vi "Update State Data.vi"(8 "error in (no error)":errorcluster, 9 "Data":variant, 10 "Argument":string, 11 "State Data":T1={"Core"={"Current VI Reference"=refnum, "Close Panel on Exit?"=FALSE}, "FP Refs"={"VI Tree"=refnum, "Window Title"=refnum, "Same as VI?"=refnum, "VI Desc"=refnum, "Help Path"=refnum, "Help Tag"=refnum, "Controls"=refnum}, "New VI Data"=[], "Saved VI Data"=[], "Current Path"=path "", "FP"={"Selected VI Data"=0, "Help Path"="", "Help Tag"="", "Help URL"="", "Help Type"=enum."Local Help File", "VI Desc"="", "Controls"=[], "Window Title"="", "Same Title?"=FALSE, "VI Tree Value"=""}, "Config Path"=path "", "Config"={"Copyright Path"=path "", "Recent Folders"=[], "Recent Files"=[], "Recent Filters"=[], "Abbreviate Names?"=FALSE, "Format Bold Tags?"=FALSE, "Show ConPane Only?"=FALSE, "Confirm Save?"=FALSE, "Confirm Revert?"=FALSE, "Confirm Save All?"=FALSE, "Confirm Revert All?"=FALSE, "Confirm Exit?"=FALSE, "Flat View?"=FALSE}, "Desc Selection"={"Selection Start"=0, "Selection End"=0}, "Displayed Indices"=[], "Filter"={"Filter Column"=enum."Description", "Filter Type"=enum."Contains", "Filter Value"="", "New Data?"=FALSE, "Enabled?"=FALSE}, "Sort"={"Sort Column"=enum."Description", "Ascending?"=FALSE, "Enabled?"=FALSE}, "Tree Map"=refnum, "VI Blacklist"={}}) -> (0 "error out":errorcluster, 3 "State Data out":T1={"Core"={"Current VI Reference"=refnum, "Close Panel on Exit?"=FALSE}, "FP Refs"={"VI Tree"=refnum, "Window Title"=refnum, "Same as VI?"=refnum, "VI Desc"=refnum, "Help Path"=refnum, "Help Tag"=refnum, "Controls"=refnum}, "New VI Data"=[], "Saved VI Data"=[], "Current Path"=path "", "FP"={"Selected VI Data"=0, "Help Path"="", "Help Tag"="", "Help URL"="", "Help Type"=enum."Local Help File", "VI Desc"="", "Controls"=[], "Window Title"="", "Same Title?"=FALSE, "VI Tree Value"=""}, "Config Path"=path "", "Config"={"Copyright Path"=path "", "Recent Folders"=[], "Recent Files"=[], "Recent Filters"=[], "Abbreviate Names?"=FALSE, "Format Bold Tags?"=FALSE, "Show ConPane Only?"=FALSE, "Confirm Save?"=FALSE, "Confirm Revert?"=FALSE, "Confirm Save All?"=FALSE, "Confirm Revert All?"=FALSE, "Confirm Exit?"=FALSE, "Flat View?"=FALSE}, "Desc Selection"={"Selection Start"=0, "Selection End"=0}, "Displayed Indices"=[], "Filter"={"Filter Column"=enum."Description", "Filter Type"=enum."Contains", "Filter Value"="", "New Data?"=FALSE, "Enabled?"=FALSE}, "Sort"={"Sort Column"=enum."Description", "Ascending?"=FALSE, "Enabled?"=FALSE}, "Tree Map"=refnum, "VI Blacklist"={}})   [LabVIEW 2020, in "VI Properties Editor.lvlib"]
doc: "Updates one or more elements of <B>State Data</B> based on <B>Argument</B> and <B>Data</B>."
uses:
  VI Properties Editor.lvlib
  Tree Map/Tree Map/Tree Map.lvclass
  <vilib>/ErrorRing/Error Ring.xnode
  3573416a-ab14-40fa-8eb1-e5c23e8662a1.vi
  6c3ab29c-e086-46da-822f-1f7a3bdde8cc.vi
  CTLs/Column Name.ctl
  CTLs/Filter Type.ctl
  c05ae38d-f8ec-456d-8819-95a6d1f6576e.vi
  <vilib>/Utility/error.llb/Error Cluster From Error Code.vi
  <vilib>/picture/picture.llb/imagedata.ctl
  CTLs/VI Properties.ctl
  CTLs/Control Properties.ctl
  CTLs/VI Data.ctl
  CTLs/Main Front Panel Controls.ctl
  CTLs/Config.ctl
  <vilib>/Utility/miscctls.llb/LVSelectionTypeDef.ctl
  CTLs/Filter Info.ctl
  CTLs/Main References.ctl
  CTLs/Main State Data.ctl
  CTLs/Sort Info.ctl
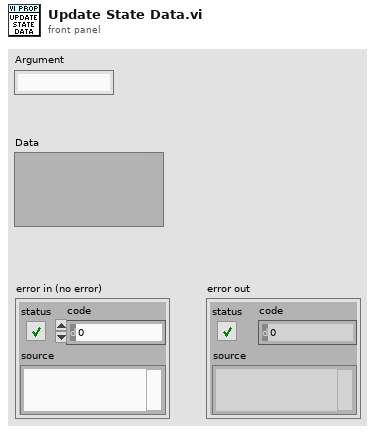
[diagram p1: front panel]
types:
  T1 = typedef "VI Properties Editor.lvlib/Main State Data.ctl" = cluster{"Core":cluster{"Current VI Reference":refnum<vi>, "Close Panel on Exit?":bool}, "FP Refs":T2, "New VI Data":T3[], "Saved VI Data":T3[], "Current Path":path, "FP":T7, "Config Path":path, "Config":T8, "Desc Selection":T12, "Displayed Indices":i32[], "Filter":T9, "Sort":T13, "Tree Map":refnum<class "Tree Map.lvclass">, "VI Blacklist":set{string}}
  T2 = typedef "VI Properties Editor.lvlib/Main References.ctl" = cluster{"VI Tree":refnum<vi>, "Window Title":refnum<vi>, "Same as VI?":refnum<vi>, "VI Desc":refnum<vi>, "Help Path":refnum<vi>, "Help Tag":refnum<vi>, "Controls":refnum<vi>}
  T3 = typedef "VI Properties Editor.lvlib/VI Data.ctl" = cluster{"VI":T4, "Ctl Properties":T6[], "Hierarchy":string}
  T4 = typedef "VI Properties Editor.lvlib/VI Properties.ctl" = cluster{"Name":string, "Path":path, "Type":enum32{"invalid VI type", "Standard VI", "Control VI", "Global VI", "Polymorphic VI", "Configuration VI", "SubSystem", "Facade VI", "Method VI", "Statechart Diagram VI"}, "Window Title":string, "Description":string, "Help Path":path, "Help Tag":string, "Help Web URL":string, "Use Web URL?":bool, "Custom Title?":bool, "Allow Debugging?":bool, "Reentrant?":bool, "Inlined?":bool, "Reentrancy Type":enum16{"Share clones between instances", "Preallocate clone for each instance"}, "Priority":enum32{"invalid priority", "background priority", "normal priority", "above normal priority", "high priority", "time critical priority", "subroutine"}, "Preferred Exec System":enum32{"invalid execution system", "user interface", "standard", "instrument i/o", "data acquisition", "other 1", "other 2", "same as caller"}, "Auto Error Handling?":bool, "Run When Opened?":bool, "Suspend When Called?":bool, "Conpane Img":T5}
  T5 = typedef "imagedata.ctl" = cluster{"image type":i32, "image depth":i32, "image":u8[], "mask":u8[], "colors":u32[], "Rectangle":cluster{"left":i16, "top":i16, "right":i16, "bottom":i16}}
  T6 = typedef "VI Properties Editor.lvlib/Control Properties.ctl" = cluster{"UID":i32, "Name":string, "Caption":string, "Description":string, "Tip Strip":string, "Is Indicator?":bool, "Is on ConPane?":bool}
  T7 = typedef "VI Properties Editor.lvlib/Main Front Panel Controls.ctl" = cluster{"Selected VI Data":i32, "Help Path":string, "Help Tag":string, "Help URL":string, "Help Type":enum16{"Local Help File", "Web-based Help"}, "VI Desc":string, "Controls":string[][], "Window Title":string, "Same Title?":bool, "VI Tree Value":string}
  T8 = typedef "VI Properties Editor.lvlib/Config.ctl" = cluster{"Copyright Path":path, "Recent Folders":path[], "Recent Files":path[], "Recent Filters":T9[], "Abbreviate Names?":bool, "Format Bold Tags?":bool, "Show ConPane Only?":bool, "Confirm Save?":bool, "Confirm Revert?":bool, "Confirm Save All?":bool, "Confirm Revert All?":bool, "Confirm Exit?":bool, "Flat View?":bool}
  T9 = typedef "VI Properties Editor.lvlib/Filter Info.ctl" = cluster{"Filter Column":T10, "Filter Type":T11, "Filter Value":string, "New Data?":bool, "Enabled?":bool}
  T10 = typedef "VI Properties Editor.lvlib/Column Name.ctl" = enum16{"Name", "Path", "Type", "Window Title", "Description", "Help Path", "Help Tag", "Custom Title?", "Reentrancy", "Inlined?", "Help URL", "Help Type", "Allow Debugging?", "Auto Error Handling?", "Run When Opened?", "Suspend When Called?", "Priority", "Preferred Exec Sytem"}
  T11 = typedef "VI Properties Editor.lvlib/Filter Type.ctl" = enum16{"Contains", "Equals", "Starts with", "Ends with", "Does not contain", "Does not equal", "Is empty", "Is not empty"}
  T12 = typedef "LVSelectionTypeDef.ctl" = cluster{"Selection Start":u32, "Selection End":u32}
  T13 = typedef "VI Properties Editor.lvlib/Sort Info.ctl" = cluster{"Sort Column":T10, "Ascending?":bool, "Enabled?":bool}
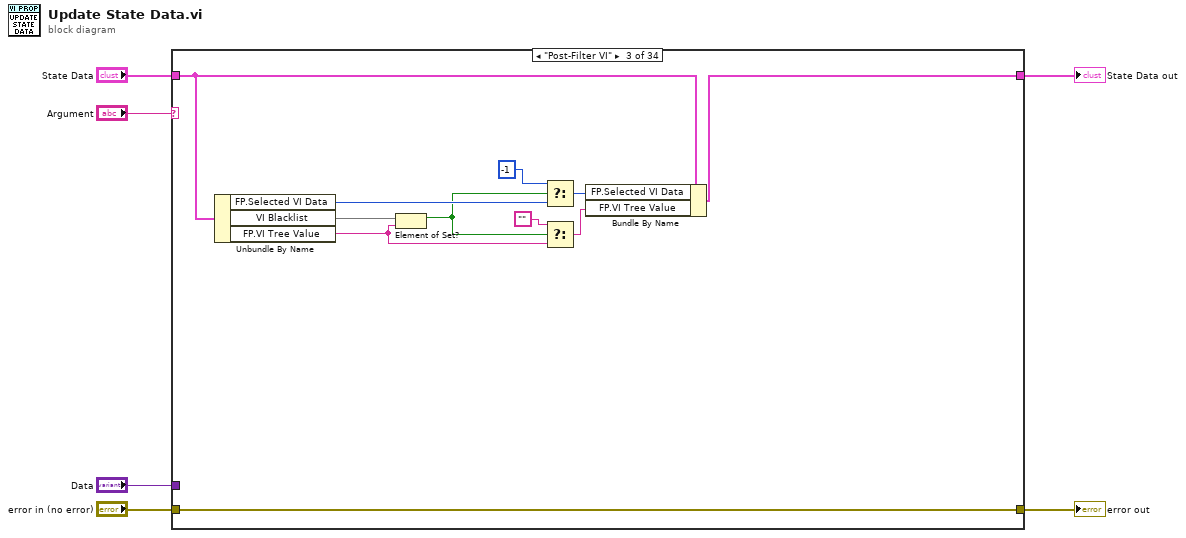
[diagram p0: block diagram]
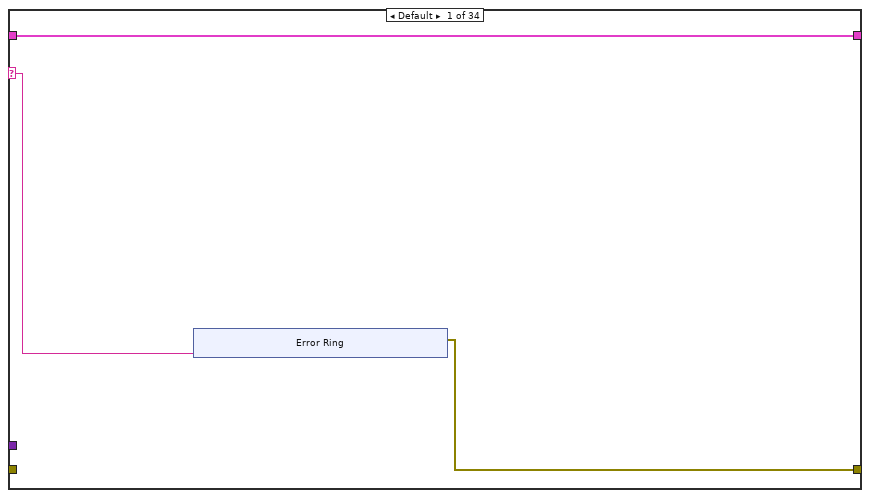
[diagram p2: hidden frame]
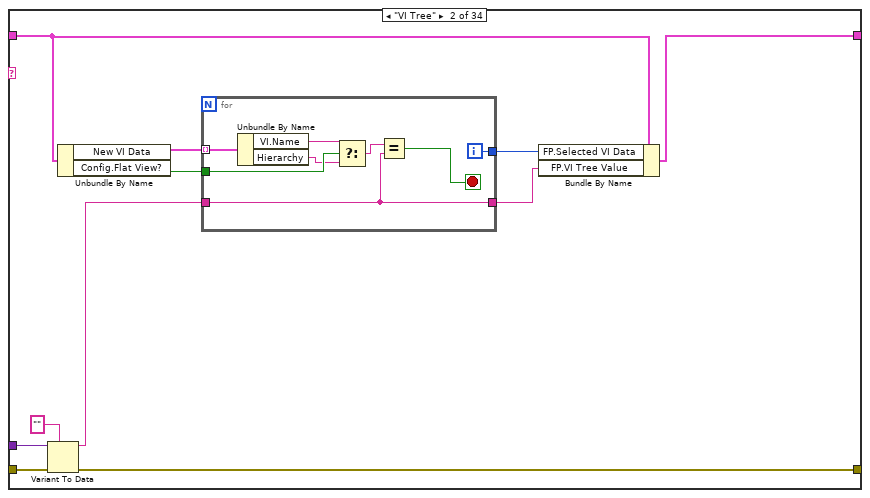
[diagram p3: hidden frame]
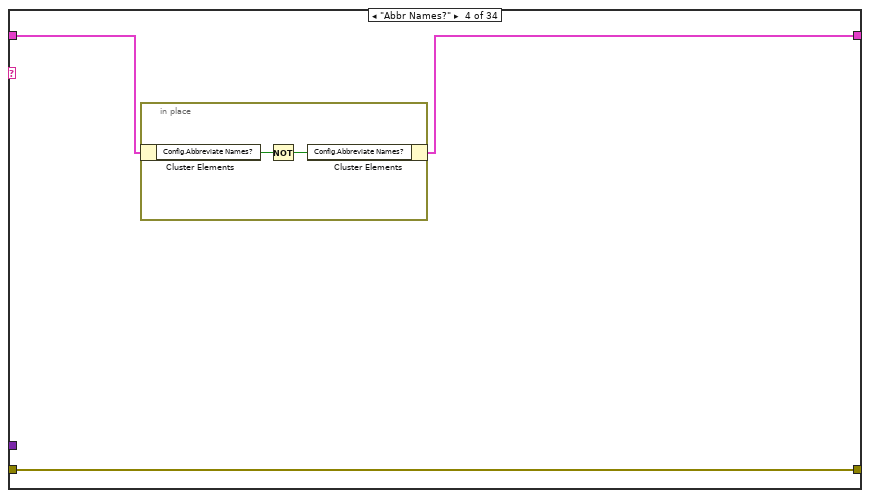
[diagram p4: hidden frame]
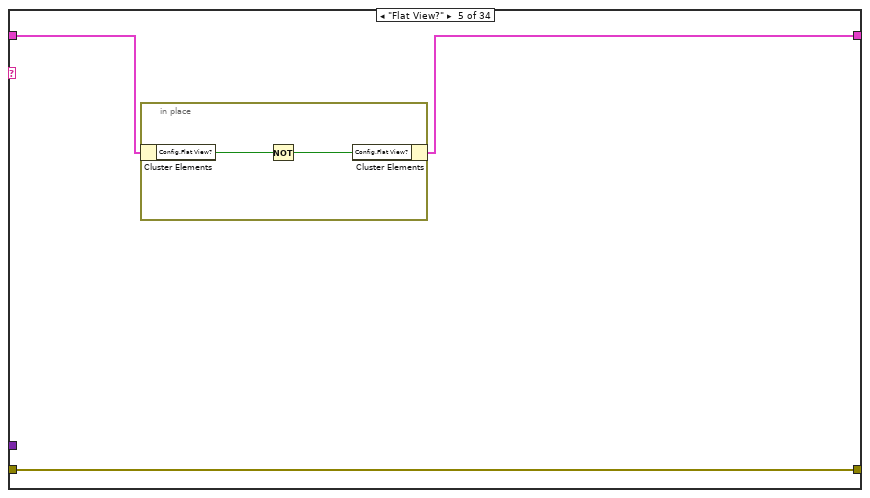
[diagram p5: hidden frame]
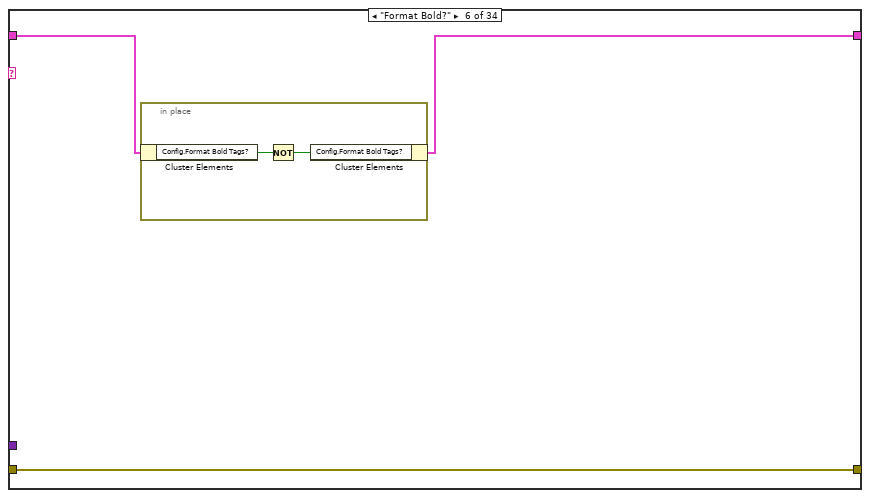
[diagram p6: hidden frame]
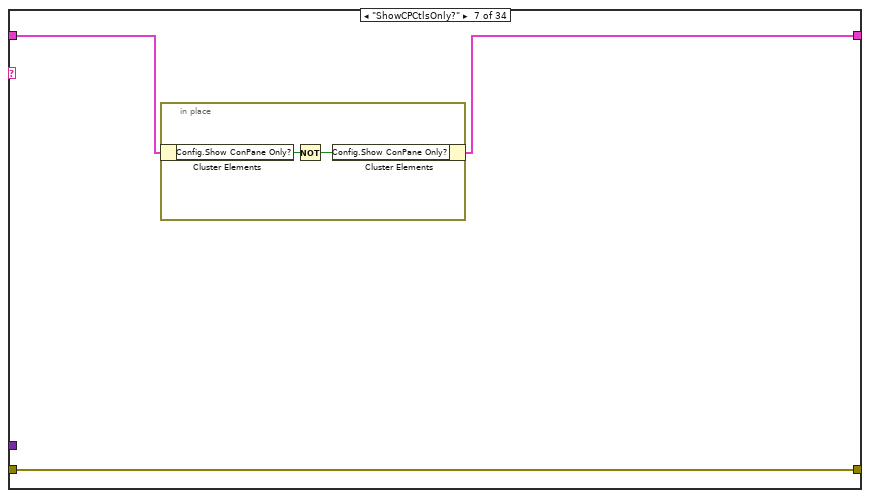
[diagram p7: hidden frame]
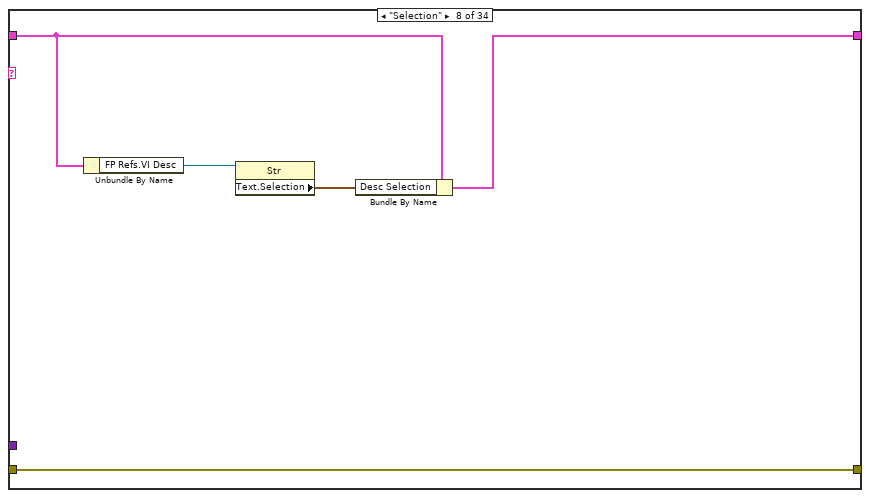
[diagram p8: hidden frame]
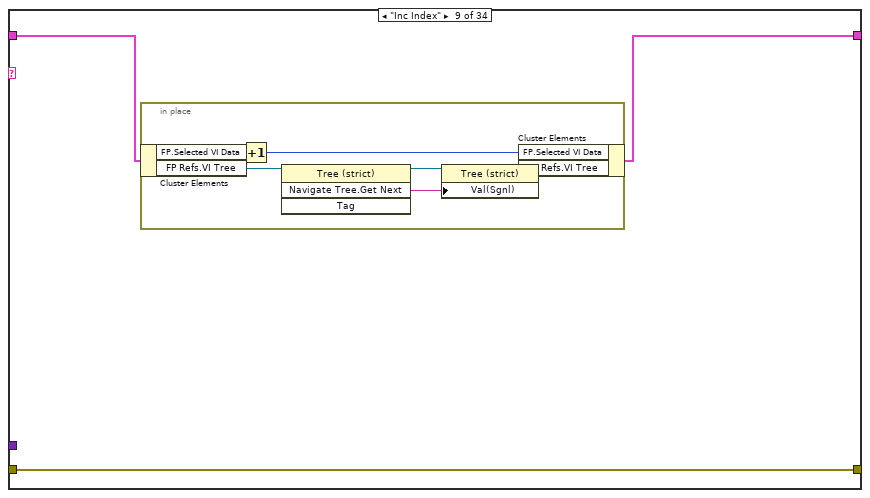
[diagram p9: hidden frame]
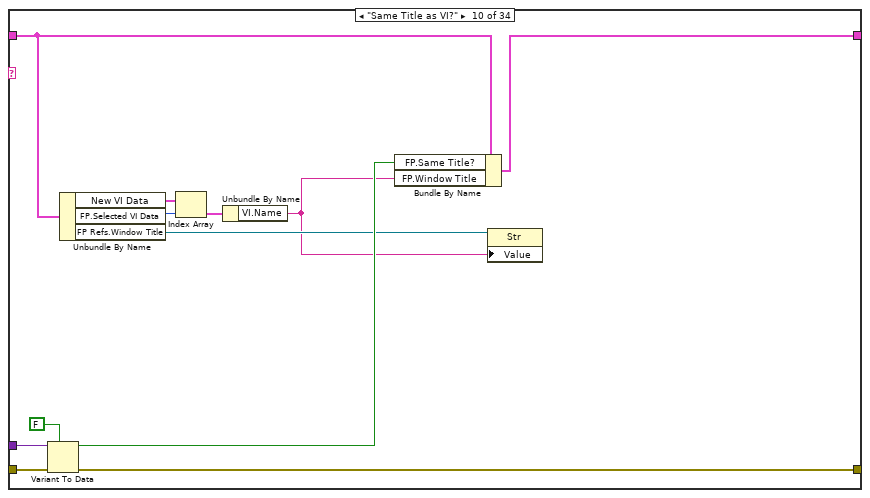
[diagram p10: hidden frame]
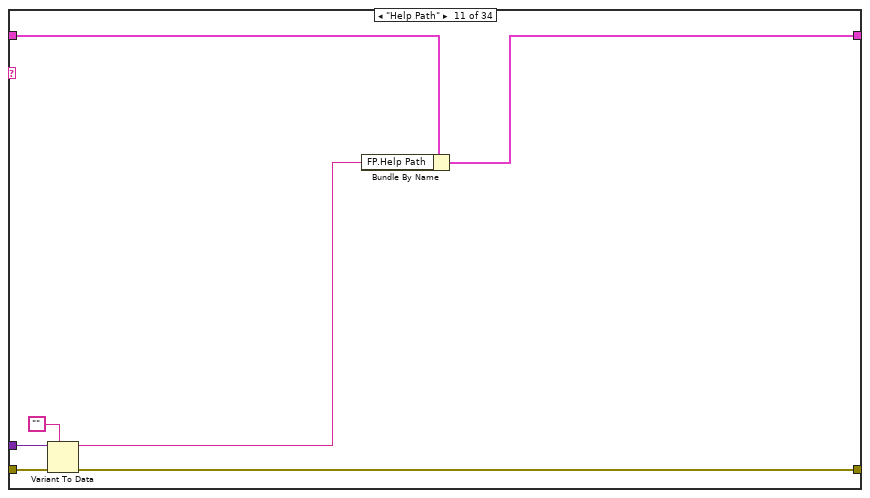
[diagram p11: hidden frame]
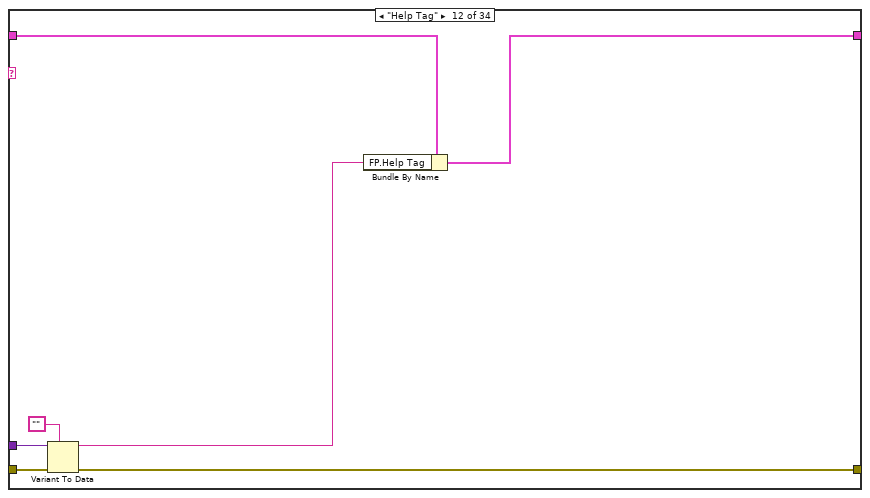
[diagram p12: hidden frame]
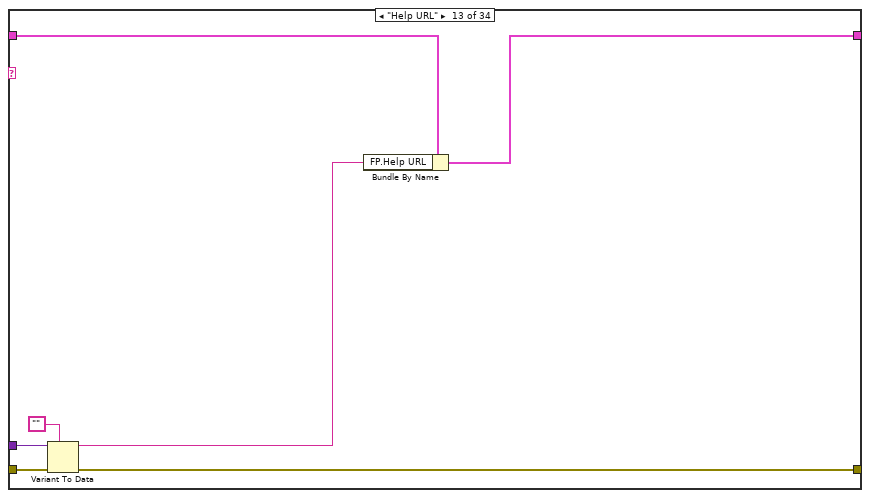
[diagram p13: hidden frame]
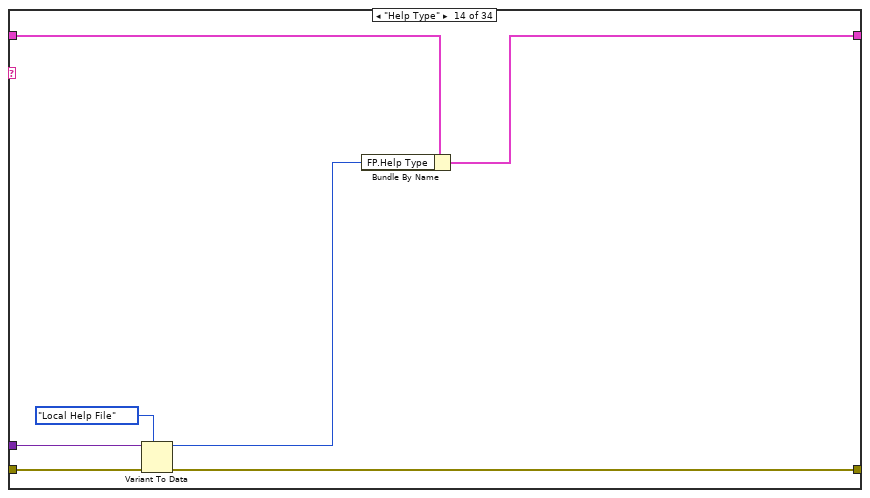
[diagram p14: hidden frame]
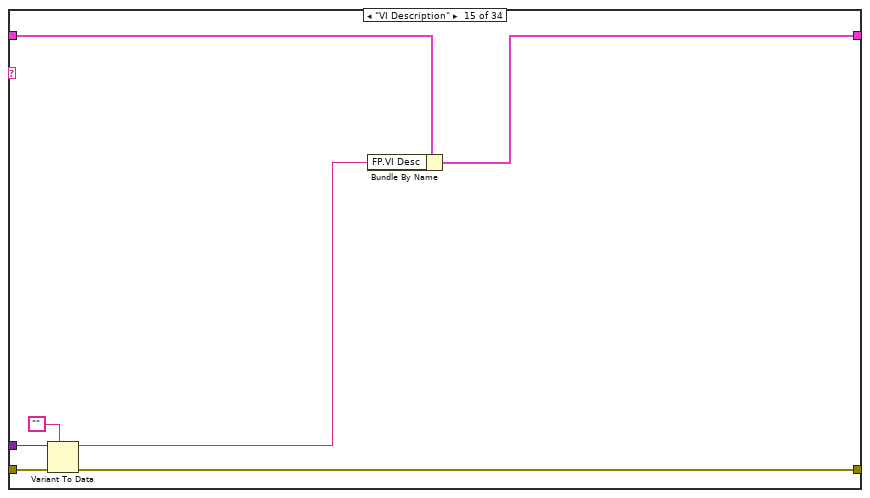
[diagram p15: hidden frame]
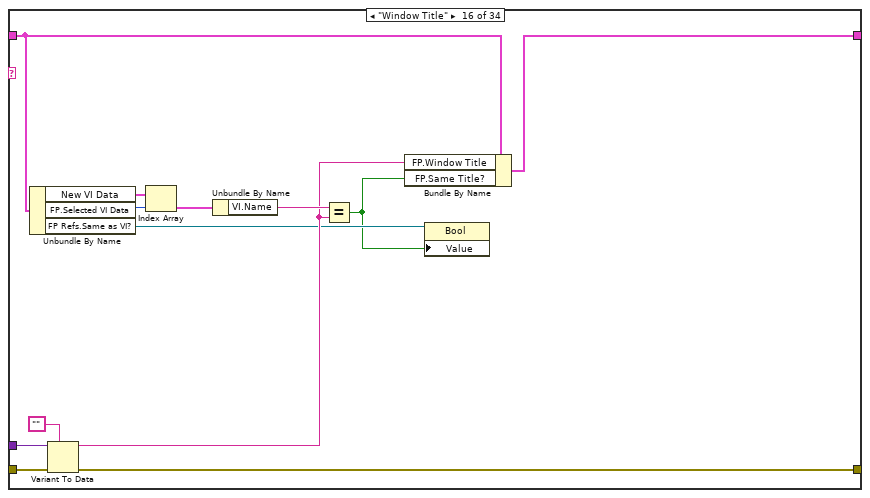
[diagram p16: hidden frame]
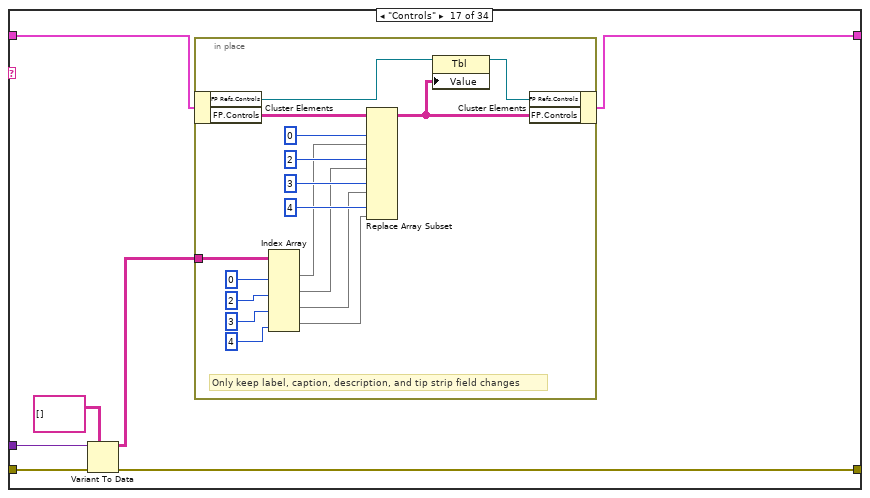
[diagram p17: hidden frame]
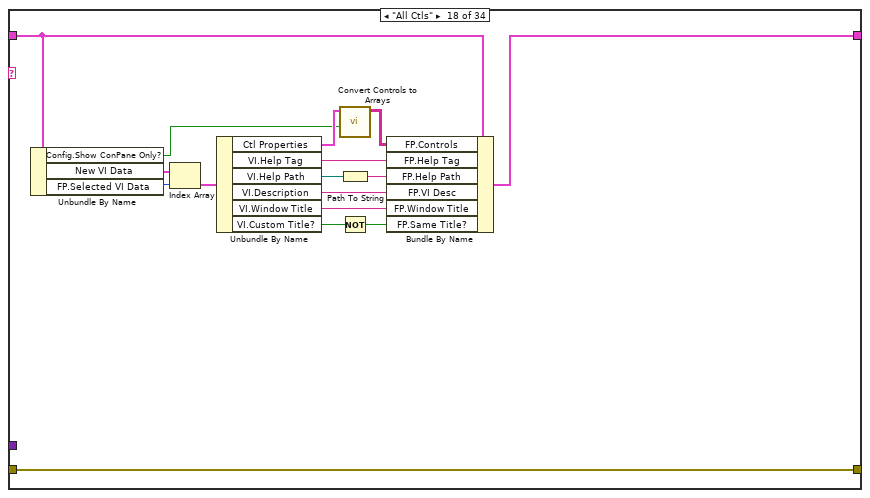
[diagram p18: hidden frame]
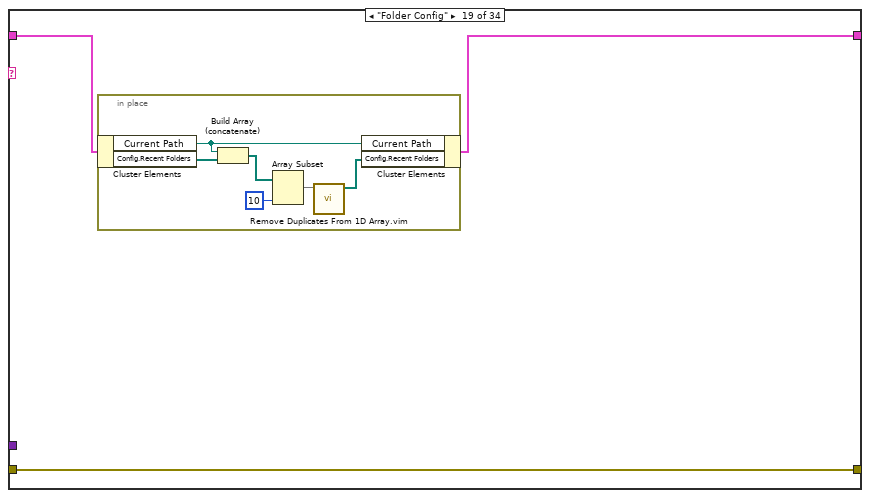
[diagram p19: hidden frame]
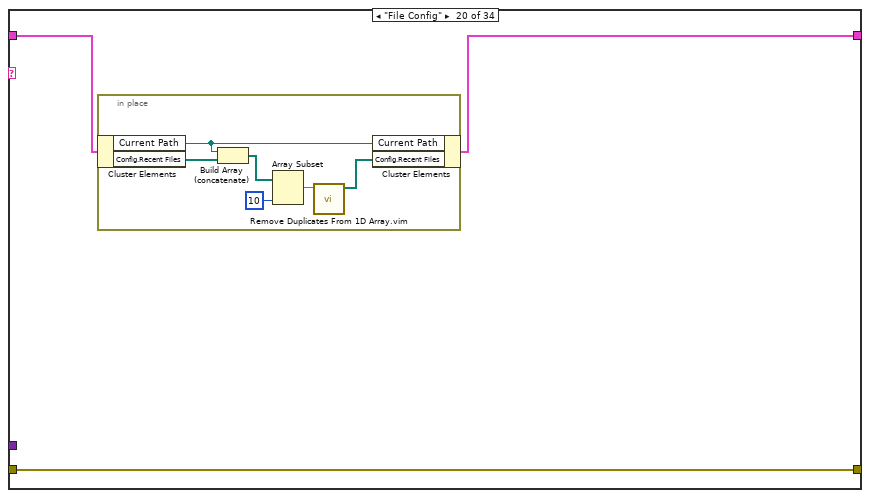
[diagram p20: hidden frame]
diagram:
  n1 = case shown="\"Post-Filter VI\"" "Argument" {
    selector: "Argument" -> [w8 _ _ _ _ _ _ _ _ _ _ _ _ _ _ _ _ _ _ _ _ w214 w224 w234 w248 w258 _ _ _ _ w293 _ _ _]
    tunnel: "error in (no error)" -> [_ w27 w44 w49 w54 w59 w64 w71 w74 w92 w99 w106 w113 w120 w127 w140 w147 w178 w183 w192 w201 w216 w226 w236 w250 w260 w266 w272 w279 w284 w295 w300 w305 w310]
    tunnel: "State Data" -> [w9 w22 w45 w48 w53 w58 w63 w68 w73 w83 w96 w103 w110 w118 w124 w133 w143 w179 w181 w190 w199 w210 w220 w230 w244 w254 w264 w270 w277 w282 w290 w298 w303 w308]
    tunnel: "Data" -> [_ w26 _ _ _ _ _ _ _ w91 w98 w105 w112 w119 w126 w139 w146 _ _ _ _ _ _ _ _ _ _ _ _ _ _ _ _ _]
    tunnel: [w7 w24 w44 w49 w54 w59 w64 w71 w74 w88 w94 w101 w108 w117 w122 w137 w145 w178 w183 w192 w201 w216 w226 w236 w250 w260 w266 w272 w279 w284 w295 w300 w305 w310] -> w1
    tunnel: [w9 w23 w46 w47 w52 w57 w62 w69 w72 w87 w93 w100 w107 w116 w121 w136 w141 w180 w182 w191 w200 w215 w225 w235 w249 w259 w265 w271 w278 w283 w294 w299 w304 w309] -> w5
    frame Default {
      n2 = xnode "Error Ring"("parameter 0"=w8) -> ("error out"=w7:errorcluster)
    }
    frame "VI Tree" {
      n3 = Variant To Data(error in=w27, type="", Variant=w26) -> (data=w19:string, error out=w24:errorcluster)
      n4 = Unbundle By Name(w22) -> ("New VI Data"=w21:T3[], "Config.Flat View?"=w17:bool)
      n5 = for {
        tunnel: w21 -> [w35] mode=indexing
        tunnel: [w34] -> w20
        tunnel: w19 -> [w32]
        tunnel: [w32] -> w18
        tunnel: w17 -> [w30]
        i -> [w34]
        stop <- w33 stop-if-true
        n6 = Unbundle By Name(w35) -> ("VI.Name"=w29:string, "Hierarchy"=w28:string)
        n7 = Select(t=w29, s=w30, f=w28) -> (s? t:f=w31:string)
        n8 = Equal?(x=w31, y=w32) -> (x = y?=w33:bool)
      }
      n9 = Bundle By Name(cluster=w22, "FP.Selected VI Data"=w20, "FP.VI Tree Value"=w18) -> (w23:T1)
    }
    frame "Post-Filter VI" {
      n10 = Unbundle By Name(w45) -> ("FP.Selected VI Data"=w40:i32, "VI Blacklist"=w42:set{string}, "FP.VI Tree Value"=w36:string)
      n11 = Element of Set?(10:w36, 11:w42) -> (3:w39:bool)
      n12 = Select(t=-1, s=w39, f=w40) -> (s? t:f=w43:i32)
      n13 = Select(t="", s=w39, f=w36) -> (s? t:f=w38:string)
      n14 = Bundle By Name(cluster=w45, "FP.Selected VI Data"=w43, "FP.VI Tree Value"=w38) -> (w46:T1)
    }
    frame "Abbr Names?" {
      n15 = in-place {
        n16 = in-place-cluster #1(w48) -> ("Config.Abbreviate Names?"=w51:bool)
        n17 = Not(x=w51) -> (.not. x?=w50:bool)
        n18 = in-place-cluster #1("Config.Abbreviate Names?"=w50) -> (w47:T1)
      }
    }
    frame "Flat View?" {
      n19 = in-place {
        n20 = in-place-cluster #2(w53) -> ("Config.Flat View?"=w56:bool)
        n21 = Not(x=w56) -> (.not. x?=w55:bool)
        n22 = in-place-cluster #2("Config.Flat View?"=w55) -> (w52:T1)
      }
    }
    frame "Format Bold?" {
      n23 = in-place {
        n24 = in-place-cluster #3(w58) -> ("Config.Format Bold Tags?"=w61:bool)
        n25 = Not(x=w61) -> (.not. x?=w60:bool)
        n26 = in-place-cluster #3("Config.Format Bold Tags?"=w60) -> (w57:T1)
      }
    }
    frame "ShowCPCtlsOnly?" {
      n27 = in-place {
        n28 = in-place-cluster #4(w63) -> ("Config.Show ConPane Only?"=w66:bool)
        n29 = Not(x=w66) -> (.not. x?=w65:bool)
        n30 = in-place-cluster #4("Config.Show ConPane Only?"=w65) -> (w62:T1)
      }
    }
    frame "Selection" {
      n31 = Unbundle By Name(w68) -> ("FP Refs.VI Desc"=w67:refnum<vi>)
      n32 = property on="Property Node" class="Str"(reference=w67) -> ("Text.Selection"=w70:T12)  [unwired: 1 in, 2 out]
      n33 = Bundle By Name(cluster=w68, "Desc Selection"=w70) -> (w69:T1)
    }
    frame "Inc Index" {
      n34 = in-place {
        n35 = in-place-cluster #5(w73) -> ("FP.Selected VI Data"=w80:i32, "FP Refs.VI Tree"=w79:refnum<vi>)
        n36 = Increment(x=w80) -> (x+1=w77:i32)
        n37 = invoke class="Tree (strict)" method="Navigate Tree.Get Next"(reference=w79) -> (reference out=w78:refnum<vi>, "Navigate Tree:Get Next Item"=w75:string)  [unwired: 3 in, 2 out]
        n38 = property class="Tree (strict)"(reference=w78, "Val(Sgnl)"=w75) -> (reference out=w76:refnum<vi>)  [unwired: 1 in, 1 out]
        n39 = in-place-cluster #5("FP.Selected VI Data"=w77, "FP Refs.VI Tree"=w76) -> (w72:T1)
      }
    }
    frame "Same Title as VI?" {
      n40 = Variant To Data(error in=w92, type=FALSE, Variant=w91) -> (data=w89:bool, error out=w88:errorcluster)
      n41 = Unbundle By Name(w83) -> ("New VI Data"=w86:T3[], "FP.Selected VI Data"=w85:i32, "FP Refs.Window Title"=w82:refnum<vi>)
      n42 = Index Array(array=w86, index=w85) -> (element=w84:T3)
      n43 = Unbundle By Name(w84) -> ("VI.Name"=w81:string)
      n44 = Bundle By Name(cluster=w83, "FP.Same Title?"=w89, "FP.Window Title"=w81) -> (w87:T1)
      n45 = property class="Str"(reference=w82, "Value"=w81) -> ()  [unwired: 1 in, 2 out]
    }
    frame "Help Path" {
      n46 = Variant To Data(error in=w99, type="", Variant=w98) -> (data=w95:string, error out=w94:errorcluster)
      n47 = Bundle By Name(cluster=w96, "FP.Help Path"=w95) -> (w93:T1)
    }
    frame "Help Tag" {
      n48 = Variant To Data(error in=w106, type="", Variant=w105) -> (data=w102:string, error out=w101:errorcluster)
      n49 = Bundle By Name(cluster=w103, "FP.Help Tag"=w102) -> (w100:T1)
    }
    frame "Help URL" {
      n50 = Variant To Data(error in=w113, type="", Variant=w112) -> (data=w109:string, error out=w108:errorcluster)
      n51 = Bundle By Name(cluster=w110, "FP.Help URL"=w109) -> (w107:T1)
    }
    frame "Help Type" {
      n52 = Variant To Data(error in=w120, type=enum16{"Local Help File", "Web-based Help"}."Local Help File" ("FP.Help Type"), Variant=w119) -> (data=w114:enum16{"Local Help File", "Web-based Help"}, error out=w117:errorcluster)
      n53 = Bundle By Name(cluster=w118, "FP.Help Type"=w114) -> (w116:T1)
    }
    frame "VI Description" {
      n54 = Variant To Data(error in=w127, type="", Variant=w126) -> (data=w123:string, error out=w122:errorcluster)
      n55 = Bundle By Name(cluster=w124, "FP.VI Desc"=w123) -> (w121:T1)
    }
    frame "Window Title" {
      n56 = Unbundle By Name(w133) -> ("New VI Data"=w135:T3[], "FP.Selected VI Data"=w134:i32, "FP Refs.Same as VI?"=w129:refnum<vi>)
      n57 = Variant To Data(error in=w140, type="", Variant=w139) -> (data=w130:string, error out=w137:errorcluster)
      n58 = Index Array(array=w135, index=w134) -> (element=w132:T3)
      n59 = Unbundle By Name(w132) -> ("VI.Name"=w131:string)
      n60 = Equal?(x=w131, y=w130) -> (x = y?=w128:bool)
      n61 = Bundle By Name(cluster=w133, "FP.Window Title"=w130, "FP.Same Title?"=w128) -> (w136:T1)
      n62 = property class="Bool"(reference=w129, "Value"=w128) -> ()  [unwired: 1 in, 2 out]
    }
    frame "Controls" {
      n63 = Variant To Data(error in=w147, type=string[][] [], Variant=w146) -> (data=w142:string[][], error out=w145:errorcluster)
      n64 = in-place {
        in-place-border: w142 -> [w163]
        # "Only keep label, caption, description, and tip strip field changes"
        n65 = in-place-cluster #6(w143) -> ("FP Refs.Controls"=w152:refnum<vi>, "FP.Controls"=w162:string[][])
        n66 = Index Array(array=w163, index (col) #1=0 ("disabled index (col)"), index (col) #2=2 ("index (row)"), index (col) #3=3 ("index (row)"), index (col) #4=4 ("index (row)")) -> (element #1=w155:string[], element #2=w154:string[], element #3=w153:string[], element #4=w148:string[])  [unwired: 4 in]
        n67 = Replace Array Subset(array=w162, new element #1=w155, index (col) #1=0 ("index (row)"), new element #2=w154, index (col) #2=2 ("index (row)"), new element #3=w153, index (col) #3=3 ("index (row)"), new element #4=w148, index (col) #4=4 ("index (row)")) -> (w150:string[][])  [unwired: 4 in]
        n68 = property class="Tbl"(reference=w152, "Value"=w150) -> (reference out=w151:refnum<vi>)  [unwired: 1 in, 1 out]
        n69 = in-place-cluster #6("FP Refs.Controls"=w151, "FP.Controls"=w150) -> (w141:T1)
      }
    }
    frame "All Ctls" {
      n70 = Unbundle By Name(w179) -> ("Config.Show ConPane Only?"=w165:bool, "New VI Data"=w177:T3[], "FP.Selected VI Data"=w176:i32)
      n71 = Index Array(array=w177, index=w176) -> (element=w175:T3)
      n72 = Unbundle By Name(w175) -> ("Ctl Properties"=w166:T6[], "VI.Help Tag"=w170:string, "VI.Help Path"=w172:path, "VI.Description"=w174:string, "VI.Window Title"=w169:string, "VI.Custom Title?"=w168:bool)
      n73 = call "Convert Controls to Arrays.vi"("ConPane Only?"=w165, "Ctl Properties"=w166) -> ("Control Array"=w173:string[][])  [unwired: 9 in]
      n74 = Path To String(path=w172) -> (string=w171:string)
      n75 = Not(x=w168) -> (.not. x?=w167:bool)
      n76 = Bundle By Name(cluster=w179, "FP.Controls"=w173, "FP.Help Tag"=w170, "FP.Help Path"=w171, "FP.VI Desc"=w174, "FP.Window Title"=w169, "FP.Same Title?"=w167) -> (w180:T1)
    }
    frame "Folder Config" {
      n77 = in-place {
        n78 = in-place-cluster #7(w181) -> ("Current Path"=w186:path, "Config.Recent Folders"=w189:path[])
        n79 = Build Array (concatenate)(w186, w189) -> (w188:path[])
        n80 = Array Subset(array=w188, length=10) -> (w185:path[])  [unwired: 1 in]
        n81 = call "Remove Duplicates From 1D Array.vim"("array"=w185) -> ("array with duplicates removed"=w184:path[])  [unwired: 10 in]
        n82 = in-place-cluster #7("Current Path"=w186, "Config.Recent Folders"=w184) -> (w182:T1)
      }
    }
    frame "File Config" {
      n83 = in-place {
        n84 = in-place-cluster #8(w190) -> ("Current Path"=w195:path, "Config.Recent Files"=w198:path[])
        n85 = Build Array (concatenate)(w195, w198) -> (w197:path[])
        n86 = Array Subset(array=w197, length=10) -> (w194:path[])  [unwired: 1 in]
        n87 = call "Remove Duplicates From 1D Array.vim"("array"=w194) -> ("array with duplicates removed"=w193:path[])  [unwired: 10 in]
        n88 = in-place-cluster #8("Current Path"=w195, "Config.Recent Files"=w193) -> (w191:T1)
      }
    }
    frame "Filter Config" {
      n89 = in-place {
        # "don't want multiple of the same filter because one was filtered on new data"
        n90 = in-place-cluster #9(w199) -> ("Filter"=w204:T9, "Config.Recent Filters"=w209:T9[])
        n91 = Bundle By Name(cluster=w204, "New Data?"=FALSE) -> (w202:T9)
        n92 = Build Array (concatenate)(w202, w209) -> (w208:T9[])
        n93 = Array Subset(array=w208, length=10) -> (w206:T9[])  [unwired: 1 in]
        n94 = call "Remove Duplicates From 1D Array.vim"("array"=w206) -> ("array with duplicates removed"=w205:T9[])  [unwired: 10 in]
        n95 = in-place-cluster #9("Filter"=w204, "Config.Recent Filters"=w205) -> (w200:T1)
      }
    }
    frame "FOLDER_0".."FOLDER_9" {
      n96 = Match Pattern(string=w214, regular expression="_") -> (after substring=w212:string)  [unwired: 1 in, 3 out]
      n97 = Decimal String To Number(string=w212) -> (number=w211:i32)  [unwired: 2 in, 1 out]
      n98 = in-place {
        in-place-border: w211 -> [w218]
        n99 = in-place-cluster #10(w210) -> ("Config.Recent Folders"=w219:path[])  [unwired: 1 out]
        n100 = Index Array(array=w219, index=w218) -> (element=w217:path)
        n101 = in-place-cluster #10("Current Path"=w217, "Config.Recent Folders"=w219) -> (w215:T1)
      }
    }
    frame "FILE_0".."FILE_9" {
      n102 = Match Pattern(string=w224, regular expression="_") -> (after substring=w222:string)  [unwired: 1 in, 3 out]
      n103 = Decimal String To Number(string=w222) -> (number=w221:i32)  [unwired: 2 in, 1 out]
      n104 = in-place {
        in-place-border: w221 -> [w228]
        n105 = in-place-cluster #11(w220) -> ("Config.Recent Files"=w229:path[])  [unwired: 1 out]
        n106 = Index Array(array=w229, index=w228) -> (element=w227:path)
        n107 = in-place-cluster #11("Current Path"=w227, "Config.Recent Files"=w229) -> (w225:T1)
      }
    }
    frame "FILTER_0".."FILTER_9" {
      n108 = Match Pattern(string=w234, regular expression="_") -> (after substring=w232:string)  [unwired: 1 in, 3 out]
      n109 = Decimal String To Number(string=w232) -> (number=w231:i32)  [unwired: 2 in, 1 out]
      n110 = in-place {
        in-place-border: w231 -> [w242]
        n111 = in-place-cluster #12(w230) -> ("Config.Recent Filters"=w243:T9[])  [unwired: 4 out]
        n112 = Index Array(array=w243, index=w242) -> (element=w241:T9)
        n113 = Unbundle By Name(w241) -> ("Filter Column"=w240:T10, "Filter Type"=w239:T11, "Filter Value"=w238:string)
        n114 = in-place-cluster #12("Config.Recent Filters"=w243, "Filter.Filter Column"=w240, "Filter.Filter Type"=w239, "Filter.Filter Value"=w238, "Filter.Enabled?"=TRUE) -> (w235:T1)
      }
    }
    frame "REM-FOLDER_0".."REM-FOLDER_9" {
      n115 = Match Pattern(string=w248, regular expression="_") -> (after substring=w246:string)  [unwired: 1 in, 3 out]
      n116 = Decimal String To Number(string=w246) -> (number=w245:i32)  [unwired: 2 in, 1 out]
      n117 = in-place {
        in-place-border: w245 -> [w252]
        n118 = in-place-cluster #13(w244) -> ("Config.Recent Folders"=w253:path[])
        n119 = Delete From Array(array=w253, index=w252) -> (array with subset deleted=w251:path[])  [unwired: 1 in, 1 out]
        n120 = in-place-cluster #13("Config.Recent Folders"=w251) -> (w249:T1)
      }
    }
    frame "REM-FILE_0".."REM-FILE_9" {
      n121 = Match Pattern(string=w258, regular expression="_") -> (after substring=w256:string)  [unwired: 1 in, 3 out]
      n122 = Decimal String To Number(string=w256) -> (number=w255:i32)  [unwired: 2 in, 1 out]
      n123 = in-place {
        in-place-border: w255 -> [w262]
        n124 = in-place-cluster #14(w254) -> ("Config.Recent Files"=w263:path[])
        n125 = Delete From Array(array=w263, index=w262) -> (array with subset deleted=w261:path[])  [unwired: 1 in, 1 out]
        n126 = in-place-cluster #14("Config.Recent Files"=w261) -> (w259:T1)
      }
    }
    frame "Filter" {
      n127 = in-place {
        n128 = in-place-cluster #15(w264) -> ()  [unwired: 3 out]
        n129 = in-place-cluster #15("Filter.Filter Column"=Column_Name."Description", "Filter.Filter Type"=Filter_Type."Is empty", "Filter.Enabled?"=TRUE) -> (w265:T1)
      }
    }
    frame "Filter 2" {
      n130 = in-place {
        n131 = in-place-cluster #16(w270) -> ()  [unwired: 4 out]
        n132 = in-place-cluster #16("Filter.Filter Value"="<[Bb]>.+</[Bb]>", "Filter.Filter Column"=Column_Name."Description", "Filter.Filter Type"=Filter_Type."Does not contain", "Filter.Enabled?"=TRUE) -> (w271:T1)
      }
    }
    frame "Filter Data Source" {
      n133 = in-place {
        n134 = in-place-cluster #17(w277) -> ("Filter.New Data?"=w281:bool)
        n135 = Not(x=w281) -> (.not. x?=w280:bool)
        n136 = in-place-cluster #17("Filter.New Data?"=w280) -> (w278:T1)
      }
    }
    frame "Clear Filter" {
      n137 = in-place {
        n138 = in-place-cluster #18(w282) -> ()  [unwired: 1 out]
        n139 = in-place-cluster #18("Filter.Enabled?"=FALSE) -> (w283:T1)
      }
    }
    frame "SORT_0".."SORT_99" {
      n140 = Match Pattern(string=w293, regular expression="_") -> (after substring=w291:string)  [unwired: 1 in, 3 out]
      n141 = Decimal String To Number(string=w291, default (0L)=u16 0 ("default (0 I32)")) -> (number=w289:u16)  [unwired: 1 in, 1 out]
      n142 = Type Cast(type=Column_Name."Name" ("Sort Column"), x=w289) -> (*(type *) &x=w287:T10)
      n143 = in-place {
        in-place-border: w287 -> [w297]
        n144 = in-place-cluster #19(w290) -> ()  [unwired: 2 out]
        n145 = in-place-cluster #19("Sort.Enabled?"=TRUE, "Sort.Sort Column"=w297) -> (w294:T1)
      }
    }
    frame "Unsort" {
      n146 = in-place {
        n147 = in-place-cluster #20(w298) -> ()  [unwired: 2 out]
        n148 = in-place-cluster #20("Sort.Sort Column"=Column_Name."Name" ("Sort Column"), "Sort.Enabled?"=FALSE) -> (w299:T1)
      }
    }
    frame "Sort Order" {
      n149 = in-place {
        n150 = in-place-cluster #21(w303) -> ("Sort.Ascending?"=w307:bool)
        n151 = Not(x=w307) -> (.not. x?=w306:bool)
        n152 = in-place-cluster #21("Sort.Ascending?"=w306) -> (w304:T1)
      }
    }
    frame "Reset VI Tree" {
      n153 = in-place {
        n154 = in-place-cluster #22(w308) -> ("FP Refs.VI Tree"=w314:refnum<vi>)  [unwired: 2 out]
        n155 = invoke class="Tree (strict)" method="Edit Tree Items.Delete"(reference=w314) -> (reference out=w313:refnum<vi>)  [unwired: 4 in, 4 out]
        n156 = in-place-cluster #22("FP.VI Tree Value"="", "FP.Selected VI Data"=-1, "FP Refs.VI Tree"=w313) -> (w309:T1)
      }
    }
  }
  "State Data out" <- w5
  "error out" <- w1
